vi "SetADcds.vi"(0 "ti gain":u32, 1 "amp":u32, 2 "ofs":i32, 3 "SHA":u8) -> ()   [LabVIEW 2014]
uses:
  ESLSCDLL.dll
panel:
  # "Init of the cds AD converter Ad9826"
  # "1=SHA mode, 0=cds mode"
  # "amplification to adjust full scale: 0..64"
  # "offset: -255..+255"
  # "only TI sensor: gain 0..255"
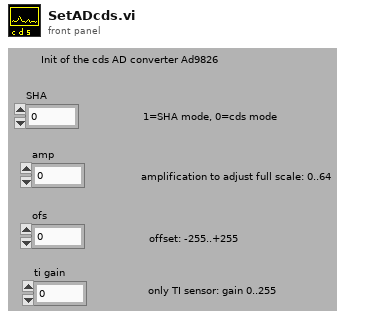
[diagram p1: front panel]
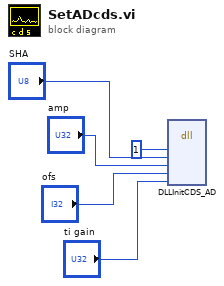
[diagram p0: block diagram]
diagram:
  n1 = dll-call lib="C:/Users/Gerhard/Documents/New64/lv/1cam/board.vis/ESLSCDLL.dll" fn="DLLInitCDS_AD" ("lwlscdll.dll:DLLRsTOREG")("drv"=u32 1, "sha"="SHA", "amp"="amp", "ofs"="ofs", "tigain"="ti gain") -> ()  [unwired: 9 in, 2 out]
